vi "ProgramControlAccess.vi"(0 "Program Interface in":refnum<class "Program Interface.lvclass">, 1 "Program Status":T1, 5 "error in (no error)":errorcluster, 8 "Robot Status":T3) -> (14 "Program Interface out":refnum<class "Program Interface.lvclass">, 19 "error out":errorcluster)   [LabVIEW 2016, in "Program Interface.lvclass"]
uses:
  Program Interface.lvclass
  Universal Robot/RobotStatus.ctl
  Universal Robot/RobotMode.ctl
  Universal Robot/OperationalMode.ctl
  Universal Robot/SafetyStatus.ctl
  Universal Robot/ProgramStatus.ctl
  Universal Robot/ProgramState.ctl
  Program Interface.lvclass/Program Interface.ctl
  Universal Robot/Universal Robot.lvclass
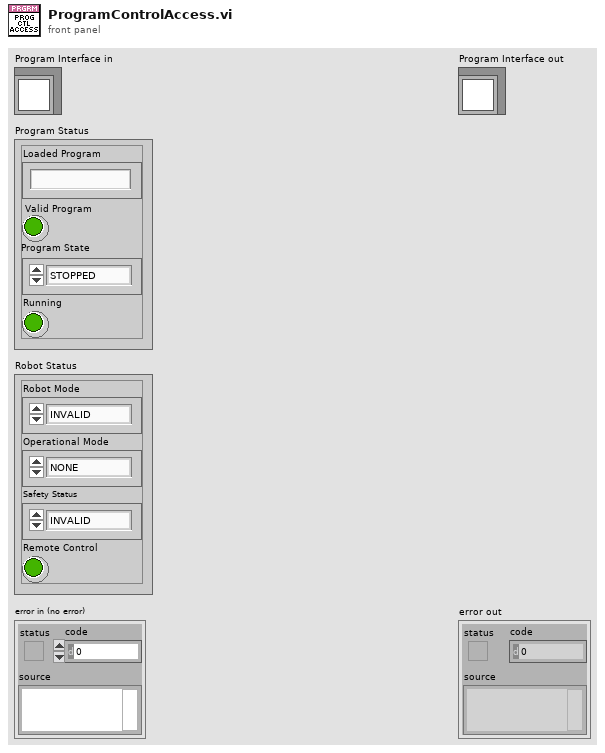
[diagram p1: front panel]
types:
  T1 = typedef "Universal Robot.lvclass/ProgramStatus.ctl" = cluster{"Loaded Program":string, "Valid Program":bool, "Program State":T2, "Running":bool}
  T2 = typedef "Universal Robot.lvclass/ProgramState.ctl" = enum16{"STOPPED", "PLAYING", "PAUSE"}
  T3 = typedef "Universal Robot.lvclass/RobotStatus.ctl" = cluster{"Robot Mode":T4, "Operational Mode":T5, "Safety Status":T6, "Remote Control":bool}
  T4 = typedef "Universal Robot.lvclass/RobotMode.ctl" = enum16{"INVALID", "NO_CONTROLLER", "DISCONNECTED", "CONFIRM_SAFETY", "BOOTING", "POWER_OFF", "POWER_ON", "IDLE", "BACKDRIVE", "RUNNING"}
  T5 = typedef "Universal Robot.lvclass/OperationalMode.ctl" = enum16{"NONE", "MANUAL", "AUTOMATIC"}
  T6 = typedef "Universal Robot.lvclass/SafetyStatus.ctl" = enum16{"INVALID", "NORMAL", "REDUCED", "PROTECTIVE_STOP", "RECOVERY", "SAFEGAURD_STOP", "SYSTEM_EMERGENCY_STOP", "ROBOT_EMERGENCY_STOP", "VIOLATION", "FAULT", "AUTOMATIC_MODE_SAFEGAURD_STOP", "SYSTEM_THREE_POSITION_ENABLING_STOP"}
  T7 = enum8{"Enabled", "Disabled", "Disabled and Grayed Out"}
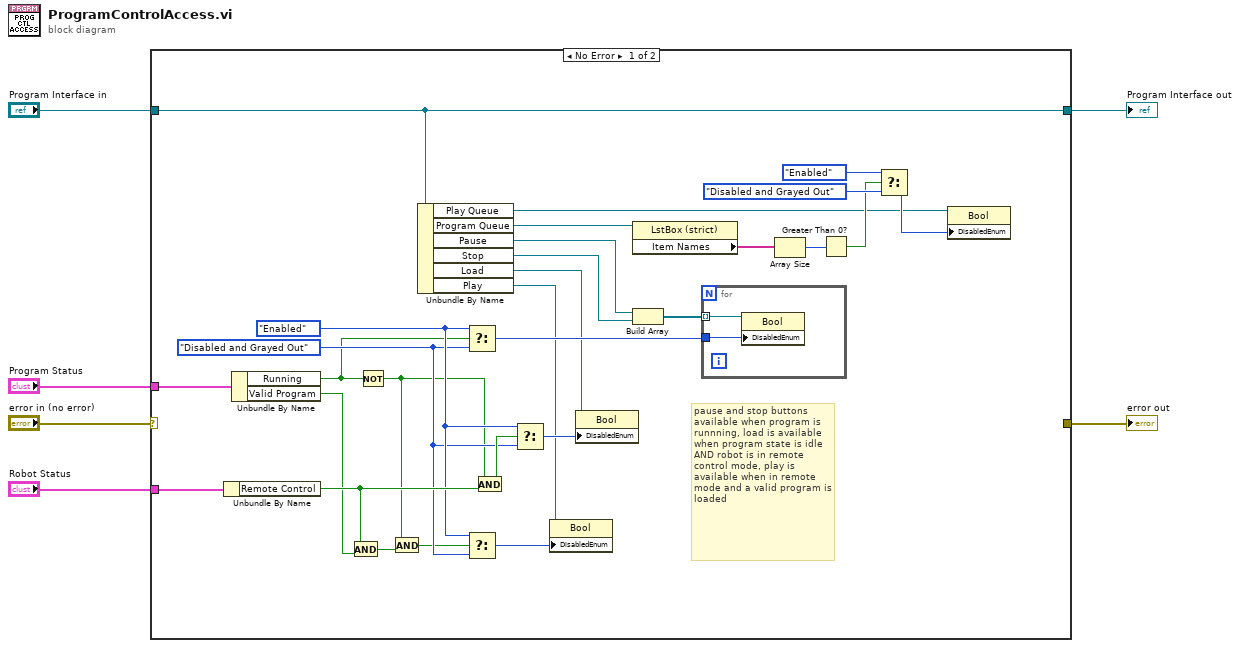
[diagram p0: block diagram]
diagram:
  n1 = case shown="No Error" "error in (no error)" {
    selector: "error in (no error)" -> [_ w38]
    tunnel: [_ w38] -> w5
    tunnel: [w34 w37] -> w3
    tunnel: "Program Interface in" -> [w34 w37]
    tunnel: "Robot Status" -> [w33 _]
    tunnel: "Program Status" -> [w27 _]
    frame No Error {
      w21 = T7."Disabled and Grayed Out" ("Disabled")
      w22 = T7."Enabled" ("Disabled")
      # "pause and stop buttons available when program is runnning, load is available when program state is idle AND robot is in remote control mode, play is available when in remote mode and a valid program is loaded"
      n2 = Unbundle By Name(w33) -> ("Remote Control"=w23:bool)
      n3 = Unbundle By Name(w27) -> ("Running"=w16:bool, "Valid Program"=w17:bool)
      n4 = And(x=w23, y=w17) -> (x .and. y?=w19:bool)
      n5 = Not(x=w16) -> (.not. x?=w15:bool)
      n6 = And(x=w15, y=w19) -> (x .and. y?=w18:bool)
      n7 = Unbundle By Name(w34) -> ("Play Queue"=w7:refnum<vi>, "Program Queue"=w14:refnum<vi>, "Pause"=w30:refnum<vi>, "Stop"=w31:refnum<vi>, "Load"=w25:refnum<vi>, "Play"=w24:refnum<vi>)
      n8 = Select(t=w22, s=w16, f=w21) -> (s? t:f=w28:T7)
      n9 = Select(t=w22, s=w18, f=w21) -> (s? t:f=w20:T7)
      n10 = And(x=w15, y=w23) -> (x .and. y?=w26:bool)
      n11 = Select(t=w22, s=w26, f=w21) -> (s? t:f=w32:T7)
      n12 = property class="Bool"(reference=w24, "DisabledEnum"=w20) -> ()  [unwired: 1 in, 2 out]
      n13 = property class="Bool"(reference=w25, "DisabledEnum"=w32) -> ()  [unwired: 1 in, 2 out]
      n14 = property class="LstBox (strict)"(reference=w14) -> ("Item Names"=w13:string[])  [unwired: 1 in, 2 out]
      n15 = Build Array(w30, w31) -> (w29:refnum<vi>[])
      n16 = for {
        tunnel: w28 -> [w36]
        tunnel: w29 -> [w35] mode=indexing
        n17 = property class="Bool"(reference=w35, "DisabledEnum"=w36) -> ()  [unwired: 1 in, 2 out]
      }
      n18 = Array Size(array=w13) -> (size(s)=w12:i32)
      n19 = Greater Than 0?(x=w12) -> (x > 0?=w9:bool)
      n20 = Select(t=T7."Enabled" ("Disabled"), s=w9, f=T7."Disabled and Grayed Out" ("Disabled")) -> (s? t:f=w8:T7)
      n21 = property class="Bool"(reference=w7, "DisabledEnum"=w8) -> ()  [unwired: 1 in, 2 out]
    }
    frame Error {
    }
  }
  "error out" <- w5
  "Program Interface out" <- w3
